vi "Add NI-XNET CAN Hardware_Add Outgoing Cyclic.vi"(6 "Cyclic Frames":T2[](array[typedef]), 8 "error in (no error)":errorcluster, 9 "ClusterName":string, 10 "Owning Database":refnum<k24>, 11 "CAN Port":refnum<k24>) -> (0 "error out":errorcluster, 3 "CAN Port out":refnum<k24>)   [LabVIEW 2019, in "Simple SysDef API.lvlib"]
uses:
  <userlib>/SimpleSysDef/Simple SysDef API.lvlib
  <userlib>/SimpleSysDef/_SubVIs/Add NI-XNET CAN Hardware_Periodic Frame Settings.ctl
  <userlib>/SimpleSysDef/_SubVIs/Add NI-XNET CAN Hardware_Frame Settings.ctl
  <userlib>/SimpleSysDef/_SubVIs/Add NI-XNET CAN Hardware_Signal Settings.ctl
  NationalInstruments.VeriStand.SystemDefinitionAPI
  <userlib>/SimpleSysDef/_SubVIs/System Definition Reference.ctl
panel:
  in  "SysDef Ref":T1
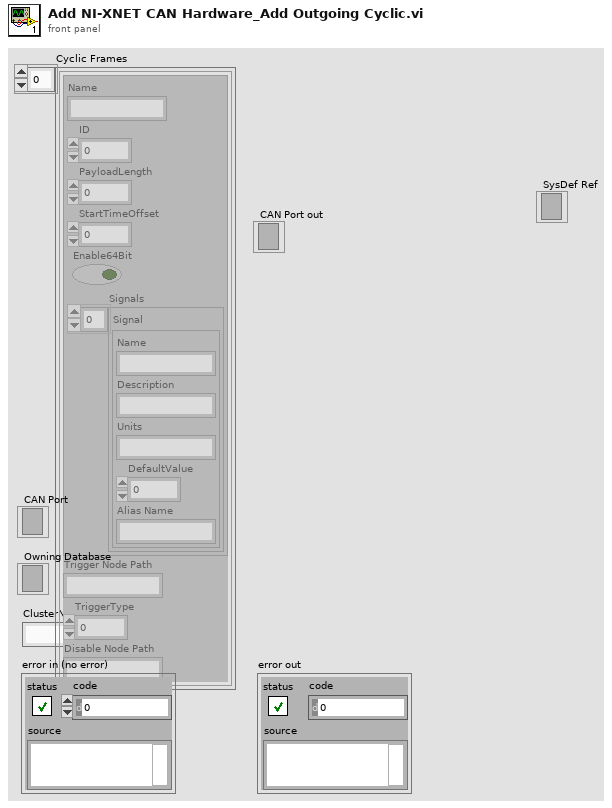
[diagram p1: front panel]
types:
  T1 = typedef "Simple SysDef API.lvlib/System Definition Reference.ctl" = refnum<k24>
  T2 = typedef "Simple SysDef API.lvlib/Add NI-XNET CAN Hardware_Periodic Frame Settings.ctl" = cluster{"Frame Settings":T3, "Trigger Node Path":string, "TriggerType":i32, "Disable Node Path":string}
  T3 = typedef "Simple SysDef API.lvlib/Add NI-XNET CAN Hardware_Frame Settings.ctl" = cluster{"Name":string, "ID":u32, "PayloadLength":u32, "StartTimeOffset":dbl, "Enable64Bit":bool, "Signals":T4[]}
  T4 = typedef "Simple SysDef API.lvlib/Add NI-XNET CAN Hardware_Signal Settings.ctl" = cluster{"Name":string, "Description":string, "Units":string, "DefaultValue":dbl, "Alias Name":string}
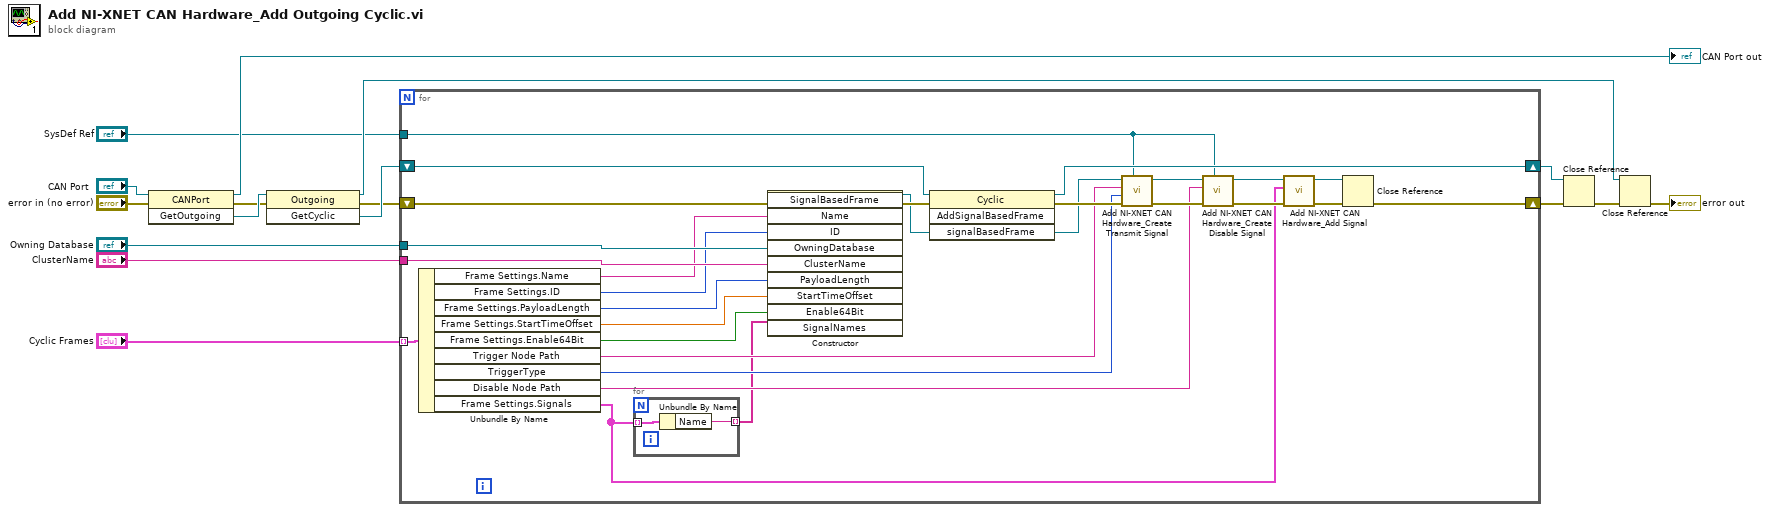
[diagram p0: block diagram]
diagram:
  n1 = invoke class="CANPort" method="GetOutgoing"(reference="CAN Port", error in="error in (no error)") -> (reference out=→"CAN Port out":refnum<k24>, error out=w7:errorcluster, "GetOutgoing"=w9:refnum<k24>)  [unwired: 1 in]
  n2 = invoke class="Outgoing" method="GetCyclic"(reference=w9, error in=w7) -> (reference out=w4:refnum<k24>, error out=w12:errorcluster, "GetCyclic"=w13:refnum<k24>)  [unwired: 1 in]
  n3 = for {
    shift-right: [w37] -> w10
    shift-left: w12 -> [w42]
    shift-right: [w38] -> w11
    shift-left: w13 -> [w41]
    tunnel: "Cyclic Frames" -> [w36] mode=indexing
    tunnel: "Owning Database" -> [w40]
    tunnel: "ClusterName" -> [w39]
    tunnel: "SysDef Ref" -> [w27]
    n4 = Unbundle By Name(w36) -> ("Frame Settings.Name"=w35:string, "Frame Settings.ID"=w34:u32, "Frame Settings.PayloadLength"=w33:u32, "Frame Settings.StartTimeOffset"=w32:dbl, "Frame Settings.Enable64Bit"=w31:bool, "Trigger Node Path"=w26:string, "TriggerType"=w25:i32, "Disable Node Path"=w24:string, "Frame Settings.Signals"=w17:T4[])
    n5 = for {
      tunnel: w17 -> [w45] mode=indexing
      tunnel: [w44] -> w18 mode=indexing
      n6 = Unbundle By Name(w45) -> ("Name"=w44:string)
    }
    n7 = constructor class="SignalBasedFrame"(error in=w42, "Name"=w35, "ID"=w34, "OwningDatabase"=w40, "ClusterName"=w39, "PayloadLength"=w33, "StartTimeOffset"=w32, "Enable64Bit"=w31, "SignalNames"=w18) -> (reference out=w23:refnum<k24>, error out=w43:errorcluster)  [unwired: 2 in, 9 out]
    n8 = invoke class="Cyclic" method="AddSignalBasedFrame"(reference=w41, error in=w43, "signalBasedFrame"=w23) -> (reference out=w38:refnum<k24>, error out=w28:errorcluster)  [unwired: 1 in, 2 out]
    n9 = call <userlib>:"Add NI-XNET CAN Hardware_Create Transmit Signal.vi"("SysDef Ref"=w27, "error in (no error)"=w28, "TriggerType"=w25, "Trigger Node Path"=w26, "Frame Based Signal"=w23) -> ("error out"=w29:errorcluster, "Frame Based Signal out"=w30:refnum<k24>)  [unwired: 5 in]
    n10 = call <userlib>:"Add NI-XNET CAN Hardware_Create Disable Signal.vi"("SysDef Ref"=w27, "error in (no error)"=w29, "Disable Node Path"=w24, "Signal Based Frame"=w30) -> ("error out"=w21:errorcluster, "Signal Based Frame out"=w22:refnum<k24>)  [unwired: 6 in]
    n11 = call <userlib>:"Add NI-XNET CAN Hardware_Add Signal.vi"("error in (no error)"=w21, "Signals"=w17, "Frame Ref"=w22) -> ("error out"=w19:errorcluster, "Frame Ref out"=w20:refnum<k24>)  [unwired: 7 in]
    n12 = Close Reference(reference=w20, error in (no error)=w19) -> (error out=w37:errorcluster)
  }
  n13 = Close Reference(reference=w11, error in (no error)=w10) -> (error out=w6:errorcluster)
  n14 = Close Reference(reference=w4, error in (no error)=w6) -> (error out=→"error out":errorcluster)
